vi "Ack Startup.vi"(8 "error in":errorcluster, 10 "Command Messenger":refnum<class "MGR.lvclass">, 11 "Starup Message":refnum<class "MSG.lvclass">) -> (0 "error out":errorcluster, 2 "Command Messenger":refnum<class "MGR.lvclass">)   [LabVIEW 2011, in "Messenging.lvlib" / "Parallel Process.lvclass"]
uses:
  Parallel Process.lvclass
  Interprocess Messenger/TextVarientMessage/MSG.lvclass
  Interprocess Messenger/TextVarientMessage/Write VarMessage.vi
  Interprocess Messenger/VarMessage/VarMessage.lvclass
  Interprocess Messenger/Messenger (Parent)/MGR.lvclass
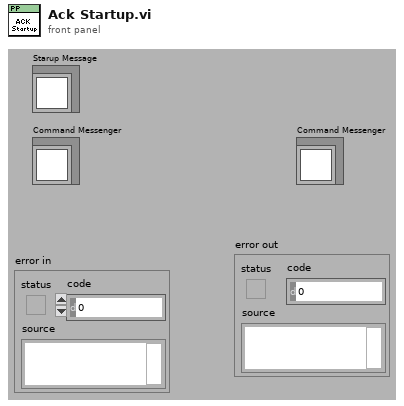
[diagram p1: front panel]
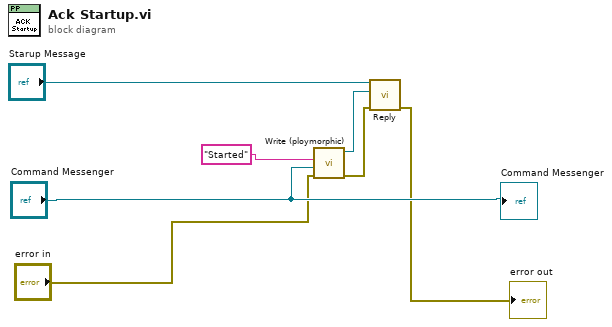
[diagram p0: block diagram]
diagram:
  n1 = call-poly "Write (ploymorphic).vi"("error in (no error)"="error in", "Varient"="Command Messenger", "Label"="Started" ("Text")) -> ("error out"=w3:errorcluster, "Message"=w5:refnum<class "VarMessage.lvclass">)  [unwired: 7 out]
  n2 = call-dynamic "Reply.vi"("error in (no error)"=w3, "Reply"=w5, "Message to Reply to"="Starup Message") -> ("error out"=→"error out":errorcluster)  [unwired: 8 out]
  "Command Messenger" <- "Command Messenger"
